vi "Add Node.vi"(8 "error in (no error)":errorcluster, 9 "coordinates":dbl[](array[numeric]), 10 "name":string, 11 "map reference in":refnum<data-value>) -> (0 "error out":errorcluster, 2 "already exists?":bool, 3 "map reference out":refnum<data-value>)   [LabVIEW 2017, in "NI_Robotics_DirectedGraphWorldMap.lvclass"]
doc: "Adds a unique point, or node, to a map at the coordinates you specify."
uses:
  <vilib>/robotics/Navigation/shared/WorldMap/DirectedGraphWorldMap/NI_Robotics_DirectedGraphWorldMap.lvclass
  <vilib>/robotics/Navigation/shared/MapNode/DirectedGraphMapNode/NI_Robotics_DirectedGraphMapNode.lvclass
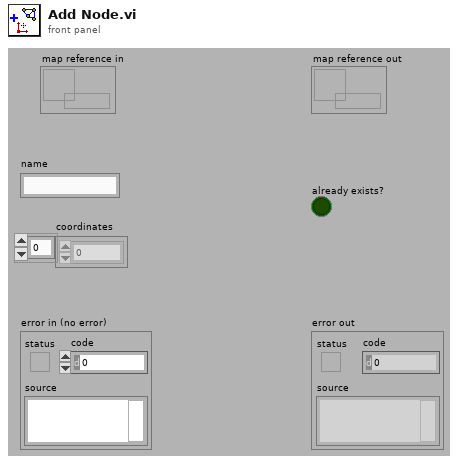
[diagram p1: front panel]
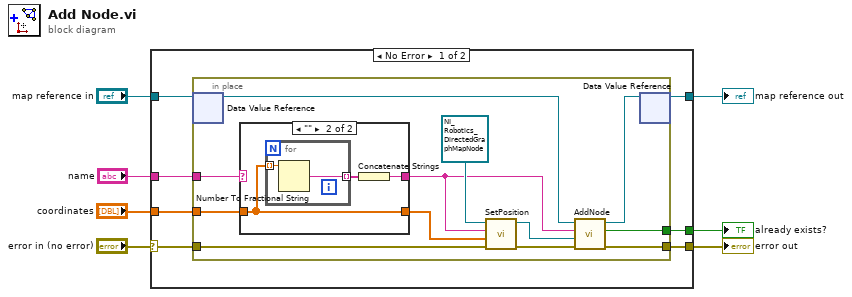
[diagram p0: block diagram]
diagram:
  n1 = case shown="No Error" "error in (no error)" {
    selector: "error in (no error)" -> [w14 w35]
    tunnel: [w13 w35] -> w6
    tunnel: "coordinates" -> [w12 _]
    tunnel: "name" -> [w11 _]
    tunnel: [w10 _] -> w3
    tunnel: "map reference in" -> [w9 w34]
    tunnel: [w8 w34] -> w1
    frame No Error {
      n2 = in-place {
        in-place-border: w14 -> [w26]
        in-place-border: [w23] -> w13
        in-place-border: w12 -> [w21]
        in-place-border: w11 -> [w20]
        in-place-border: [w17] -> w10
        n3 = in-place-dvr #1(w9) -> (w16:refnum<class "NI_Robotics_DirectedGraphWorldMap.lvclass">)  [unwired: 1 out]
        n4 = case shown="\"\"" w20 {
          selector: w20 -> [w28 _]
          tunnel: w21 -> [w27 w29]
          tunnel: [w28 w30] -> w19
          tunnel: [w27 w29] -> w18
          frame Default {
          }
          frame "" {
            n5 = for {
              tunnel: w29 -> [w33] mode=indexing
              tunnel: [w32] -> w31 mode=indexing
              n6 = Number To Fractional String(number=w33) -> (F-format string=w32:string)  [unwired: 3 in]
            }
            n7 = Concatenate Strings(w31) -> (w30:string)
          }
        }
        n8 = call-dynamic "SetPosition.vi"("error in (no error)"=w26, "coordinates"=w18, "name"=w19, "DirectedGraphMapNode in"=refnum<class "NI_Robotics_DirectedGraphMapNode.lvclass"> refnum ("DirectedGraphMapNode.lvclass")) -> ("error out"=w24:errorcluster, "DirectedGraphMapNode out"=w25:refnum<class "NI_Robotics_DirectedGraphMapNode.lvclass">)  [unwired: 6 in]
        n9 = call-dynamic "AddNode.vi"("error in (no error)"=w24, "DirectedGraphMapNode.lvclass"=w25, "Name"=w19, "DirectedGraphWorldMap in"=w16) -> ("error out"=w23:errorcluster, "Already exists"=w17:bool, "DirectedGraphWorldMap out"=w15:refnum<class "NI_Robotics_DirectedGraphWorldMap.lvclass">)  [unwired: 5 in]
        n10 = in-place-dvr #1(w15) -> (w8:refnum<data-value>)  [unwired: 1 out]
      }
    }
    frame Error {
    }
  }
  "error out" <- w6
  "already exists?" <- w3
  "map reference out" <- w1
